vi "Initialization VI.vi"(8 "error in (no error)":errorcluster, 10 "Custom XML":string, 11 "Device Item Ref in":T1 format="%.0x") -> (0 "error out":errorcluster, 3 "Device Item Ref out":T1 format="%.0x")   [LabVIEW 2016, in "UDP Sender System Explorer.lvlib"]
uses:
  UDP Sender System Explorer.lvlib
  <vilib>/NI Veristand/Custom Device API/Custom Device API.lvlib
  Channel 1.vi
  Channel 2.vi
  Section 1.vi
  <vilib>/NI Veristand/Custom Device API/Custom Device Item Ref.ctl
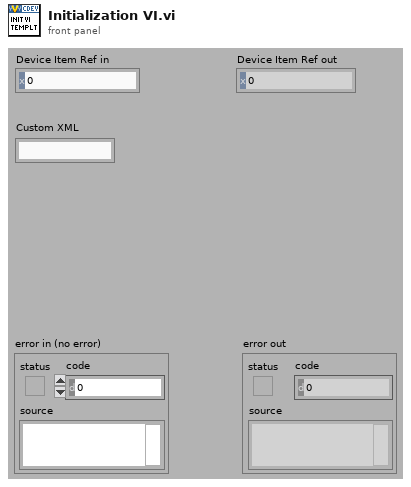
[diagram p1: front panel]
types:
  T1 = typedef "Custom Device API.lvlib/Custom Device Item Ref.ctl" = u64
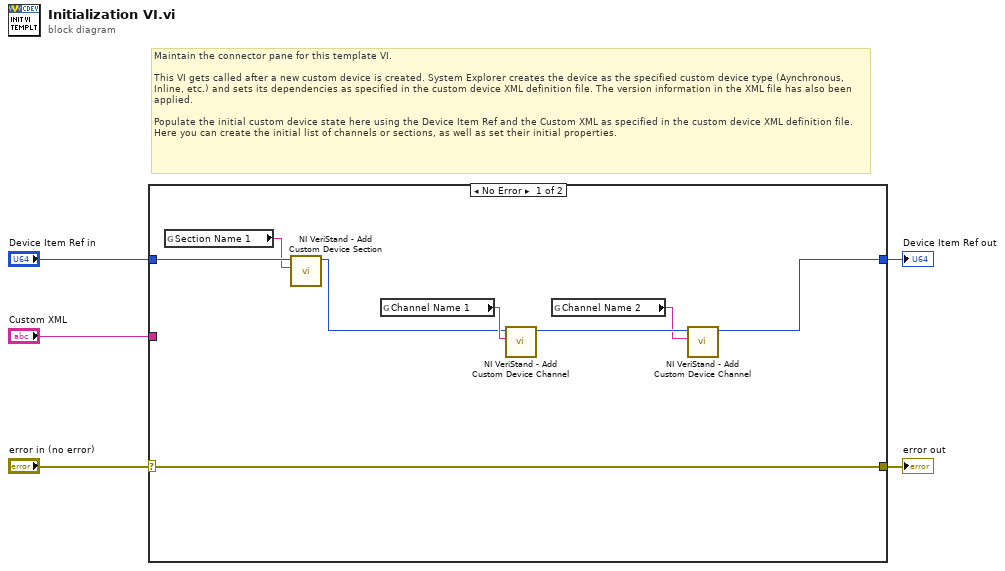
[diagram p0: block diagram]
diagram:
  # "Maintain the connector pane for this template VI.\n\nThis VI gets called after a new custom device is created. System Explorer creates the device as the specified custom device type (Aynchronous, Inline, etc.) and sets its dependencies as specified in the custom device XML definition file. The version information in the XML file has also been applied.\n\nPopulate the initial custom device state here using the Device Item Ref and the Custom XML as specified in the custom device XML definition file. Here you can create the initial list of channels or sections, as well as set their initial properties."
  n1 = case shown="No Error" "error in (no error)" {
    selector: "error in (no error)" -> [w13 w15]
    tunnel: [w13 w15] -> w5
    tunnel: [w9 w14] -> w3
    tunnel: "Device Item Ref in" -> [w8 w14]
    tunnel: "Custom XML" -> [_ _]
    frame No Error {
      n2 = global read "Section 1.vi" "Section Name 1"() -> (w6:string)
      n3 = call <vilib>:"NI VeriStand - Add Custom Device Section.vi"("Section Name"=w6, "Parent Ref in"=w8) -> ("Parent Ref out"=w7:T1)  [unwired: 6 in, 3 out]
      n4 = global read "Channel 1.vi" "Channel Name 1"() -> (w12:string)
      n5 = call <vilib>:"NI VeriStand - Add Custom Device Channel.vi"("Channel Name"=w12, "Parent Ref in"=w7) -> ("Parent Ref out"=w11:T1)  [unwired: 6 in, 3 out]
      n6 = global read "Channel 2.vi" "Channel Name 2"() -> (w10:string)
      n7 = call <vilib>:"NI VeriStand - Add Custom Device Channel.vi"("Channel Name"=w10, "Parent Ref in"=w11) -> ("Parent Ref out"=w9:T1)  [unwired: 6 in, 3 out]
    }
    frame Error {
    }
  }
  "error out" <- w5
  "Device Item Ref out" <- w3
